vi "Add Buffers.vi"(6 "Decimation":u64, 7 "Transfer Group Status":refnum<class "Status.lvclass">, 8 "error in (no error)":errorcluster, 9 "Buffers":refnum<class "Buffers.lvclass">, 10 "parent tag":string, 11 "Application Data In":T1) -> (0 "error out":errorcluster, 3 "Application Data out":T1)   [LabVIEW 2017, in "DSF Core.lvlib"]
uses:
  DSF Core.lvlib
  Main VI/Application Data.ctl
  <vilib>/NI/Memory Manager/Classes/Pointer/Pointer.lvclass
  Classes/Framework/Framework.lvclass
  Buffer Reader/Buffer Data.ctl
  Classes/Buffer/Buffer.lvclass
  C:/Program Files (x86)/National Instruments/LabVIEW 2017/vi.lib/NI/Memory Manager/Classes/Pointer/Pointer.lvclass
  Classes/Transfer Group Status/Status.lvclass
  Typedefs/DSF Engine Framework Configuration.ctl
  Typedefs/DSF Engine Plugin Configuration.ctl
  Typedefs/DSF Timing Info.ctl
  Typedefs/DSF Engine Plugin Thread Configuration.ctl
  Typedefs/DSF Settings Info.ctl
  Typedefs/DSF Engine Transfer Group Configuration.ctl
  Typedefs/DSF Direction.ctl
  Typedefs/DSF Engine Transfer Configuration.ctl
  Typedefs/DSF Byte Order.ctl
  Typedefs/DSF Engine Channel Configuration.ctl
  Typedefs/DSF Data Type.ctl
  Typedefs/DSF Timeout Behavior.ctl
  Classes/Buffers/Buffers.lvclass
  ID to Tree Items/Tree Item Type.ctl
  Classes/Buffers/Buffers.lvclass/Buffers.ctl
  <vilib>/NI/Memory Manager/Classes/Pointer/Pointer.lvclass/Pointer.ctl
  Classes/Buffer/Get Buffer Size.vi
  <vilib>/NI/Memory Manager/Classes/Pointer/Get Size.vi
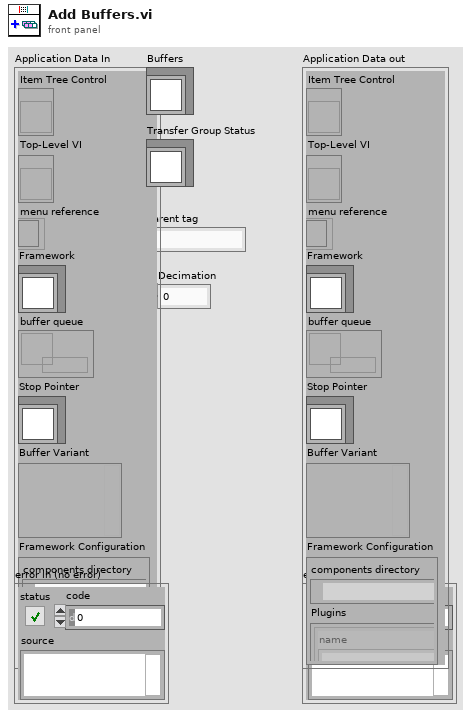
[diagram p1: front panel]
types:
  T1 = typedef "DSF Core.lvlib/Application Data.ctl" = cluster{"Item Tree Control":refnum<vi>, "Top-Level VI":refnum<vi>, "menu reference":refnum<k9>, "Framework":refnum<class "Framework.lvclass">, "buffer queue":refnum<queue>, "Stop Pointer":refnum<class "Pointer.lvclass">, "Buffer Variant":variant, "Framework Configuration":T2}
  T2 = typedef "DSF Core.lvlib/DSF Engine Framework Configuration.ctl" = cluster{"components directory":path, "Plugins":T3[]}
  T3 = typedef "DSF Core.lvlib/DSF Engine Plugin Configuration.ctl" = cluster{"name":string, "components":string[], "cycle timing":T4, "threads":T5[], "Transfer Groups":T7[], "settings":T6}
  T4 = typedef "DSF Core.lvlib/DSF Timing Info.ctl" = cluster{"priority":u64, "decimation":u64, "offset":u64}
  T5 = typedef "DSF Core.lvlib/DSF Engine Plugin Thread Configuration.ctl" = cluster{"buffer converter settings":T6, "transceiver settings":T6, "processor":i32, "priority offset":i16}
  T6 = typedef "DSF Core.lvlib/DSF Settings Info.ctl" = cluster{"key":string, "value":string}[]
  T7 = typedef "DSF Core.lvlib/DSF Engine Transfer Group Configuration.ctl" = cluster{"name":string, "direction":T8, "cycle timing":T4, "thread index":i32, "settings":T6, "Transfers":T9[], "timeout behavior":T13}
  T8 = typedef "DSF Core.lvlib/DSF Direction.ctl" = enum8{"Tx", "Rx"}
  T9 = typedef "DSF Core.lvlib/DSF Engine Transfer Configuration.ctl" = cluster{"name":string, "byte order":T10, "settings":T6, "channels":T11[]}
  T10 = typedef "DSF Core.lvlib/DSF Byte Order.ctl" = enum8{"big-endian", "little-endian"}
  T11 = typedef "DSF Core.lvlib/DSF Engine Channel Configuration.ctl" = cluster{"string offset":u64, "string data type":T12, "engine data type":T12, "name":string, "settings":T6}
  T12 = typedef "DSF Core.lvlib/DSF Data Type.ctl" = enum8{"Bool", "SGL", "DBL", "I8", "I16", "I32", "I64", "U8", "U16", "U32", "U64"}
  T13 = typedef "DSF Core.lvlib/DSF Timeout Behavior.ctl" = enum8{"Increment Late Count", "Throw Error"}
  T14 = typedef "DSF Core.lvlib/Buffer Data.ctl" = cluster{"Buffer":refnum<class "Buffer.lvclass">, "Status":refnum<class "Status.lvclass">, "decimation":u64, "avg bandwidth":dbl}
  T15 = typedef "DSF Core.lvlib/Tree Item Type.ctl" = enum16{"Framework", "Plugin Group", "Plugin", "Group", "Transfer", "Buffer", "Channel"}
  T16 = typedef "DSF Core.lvlib/Tree Item.ctl" = cluster{"Left Cell String":string, "Child Text":string[], "Child Tag":string, "Glyph Index":i32}
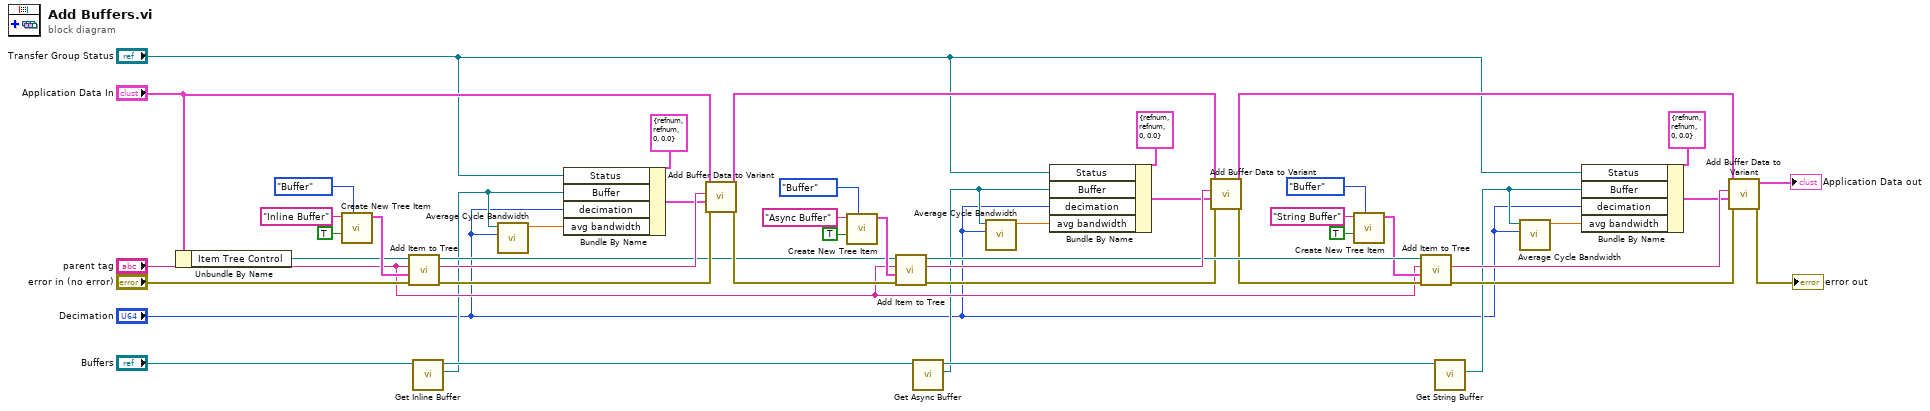
[diagram p0: block diagram]
diagram:
  n1 = Unbundle By Name("Application Data In") -> ("Item Tree Control"=w10:refnum<vi>)
  n2 = call "Create New Tree Item.vi"("Item Type"=Tree_Item_Type."Buffer", "found?"=TRUE, "Left Cell String"="Inline Buffer") -> ("Item"=w13:T16)  [unwired: 7 in, 1 out]
  n3 = call "Add Item to Tree.vi"("error in (no error)"="error in (no error)", "Item"=w13, "parent tag"="parent tag", "TreeControl in"=w10) -> ("error out"=w31:errorcluster, "new item tag"=w45:string, "TreeControl out"=w25:refnum<vi>)  [unwired: 5 in]
  n4 = call "Get Inline Buffer.vi"("Buffers in"="Buffers") -> ("Inline Buffer"=w6:refnum<class "Buffer.lvclass">, "Buffers out"=w20:refnum<class "Buffers.lvclass">)  [unwired: 9 in]
  n5 = call "Average Cycle Bandwidth.vi"("Decimation"="Decimation", "Buffer"=w6) -> ("avergage cycle bandwidth"=w7:dbl)  [unwired: 9 in]
  n6 = Bundle By Name(cluster=T14 {"Buffer"=refnum, "Status"=refnum, "decimation"=0, "avg bandwidth"=0.0} ("Buffer data"), "Status"="Transfer Group Status", "Buffer"=w6, "decimation"="Decimation", "avg bandwidth"=w7) -> (w30:T14)
  n7 = call "Add Buffer Data to Variant.vi"("error in (no error)"=w31, "Buffer data"=w30, "tag"=w45, "Application Data In in"="Application Data In") -> ("error out"=w32:errorcluster, "Application Data In out"=w35:T1)  [unwired: 6 in]
  n8 = call "Create New Tree Item.vi"("Item Type"=Tree_Item_Type."Buffer", "found?"=TRUE, "Left Cell String"="Async Buffer") -> ("Item"=w26:T16)  [unwired: 7 in, 1 out]
  n9 = call "Add Item to Tree.vi"("error in (no error)"=w32, "Item"=w26, "parent tag"="parent tag", "TreeControl in"=w25) -> ("error out"=w36:errorcluster, "new item tag"=w46:string, "TreeControl out"=w38:refnum<vi>)  [unwired: 5 in]
  n10 = call "Get Async Buffer.vi"("Buffers in"=w20) -> ("Async Buffer"=w5:refnum<class "Buffer.lvclass">, "Buffers out"=w12:refnum<class "Buffers.lvclass">)  [unwired: 9 in]
  n11 = call "Average Cycle Bandwidth.vi"("Decimation"="Decimation", "Buffer"=w5) -> ("avergage cycle bandwidth"=w4:dbl)  [unwired: 9 in]
  n12 = Bundle By Name(cluster=T14 {"Buffer"=refnum, "Status"=refnum, "decimation"=0, "avg bandwidth"=0.0} ("Buffer data"), "Status"="Transfer Group Status", "Buffer"=w5, "decimation"="Decimation", "avg bandwidth"=w4) -> (w34:T14)
  n13 = call "Add Buffer Data to Variant.vi"("error in (no error)"=w36, "Buffer data"=w34, "tag"=w46, "Application Data In in"=w35) -> ("error out"=w37:errorcluster, "Application Data In out"=w41:T1)  [unwired: 6 in]
  n14 = call "Create New Tree Item.vi"("Item Type"=Tree_Item_Type."Buffer", "found?"=TRUE, "Left Cell String"="String Buffer") -> ("Item"=w27:T16)  [unwired: 7 in, 1 out]
  n15 = call "Add Item to Tree.vi"("error in (no error)"=w37, "Item"=w27, "parent tag"="parent tag", "TreeControl in"=w38) -> ("error out"=w43:errorcluster, "new item tag"=w47:string)  [unwired: 5 in, 1 out]
  n16 = call "Get String Buffer.vi"("Buffers in"=w12) -> ("String Buffer"=w2:refnum<class "Buffer.lvclass">)  [unwired: 9 in, 1 out]
  n17 = call "Average Cycle Bandwidth.vi"("Decimation"="Decimation", "Buffer"=w2) -> ("avergage cycle bandwidth"=w3:dbl)  [unwired: 9 in]
  n18 = Bundle By Name(cluster=T14 {"Buffer"=refnum, "Status"=refnum, "decimation"=0, "avg bandwidth"=0.0} ("Buffer data"), "Status"="Transfer Group Status", "Buffer"=w2, "decimation"="Decimation", "avg bandwidth"=w3) -> (w40:T14)
  n19 = call "Add Buffer Data to Variant.vi"("error in (no error)"=w43, "Buffer data"=w40, "tag"=w47, "Application Data In in"=w41) -> ("error out"=→"error out":errorcluster, "Application Data In out"=→"Application Data out":T1)  [unwired: 6 in]
